vi "Main.vi"() -> (0 "error out":errorcluster)   [LabVIEW 2022 SP3, in "VideoMux.lvlib" / "VideoMux.lvclass"]
uses:
  VideoMux.lvclass
  VideoMux.lvclass/VideoMux.ctl
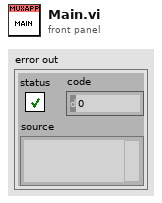
[diagram p1: front panel]
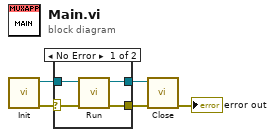
[diagram p0: block diagram]
diagram:
  n1 = call "Init.vi"() -> ("error out"=w5:errorcluster, "VideoMux out"=w4:refnum<class "VideoMux.lvclass">)  [unwired: 10 in]
  n2 = case shown="No Error" w5 {
    selector: w5 -> [w8 w10]
    tunnel: w4 -> [w9 w11]
    tunnel: [w7 w10] -> w3
    tunnel: [w6 w11] -> w2
    frame No Error {
      n3 = call "Run.vi"("error in (no error)"=w8, "VideoMux in"=w9) -> ("error out"=w7:errorcluster, "VideoMux out"=w6:refnum<class "VideoMux.lvclass">)  [unwired: 8 in]
    }
    frame Error {
    }
  }
  n4 = call "Close.vi"("error in (no error)"=w3, "VideoMux in"=w2) -> ("error out"=→"error out":errorcluster)  [unwired: 9 in]
